vi "dvp Vi Get Frame.vi"(6 "timeout":u32, 7 "piHeight":i32, 9 "piWidth":i32, 10 "pbits":u32(ring) items=["BITS_8", "BITS_10", "BITS_12", "BITS_14", "BITS_16"], 11 "handle":u32) -> (1 "piWidth out":i32, 2 "pbits out":u32(ring) items=["BITS_8", "BITS_10", "BITS_12", "BITS_14", "BITS_16"], 3 "function return":string, 5 "piHeight out":i32)   [LabVIEW 2018, in "LabViewDVPCamera.lvlib"]
doc: "LabviewDvp2Api char* dvpViGetFrame(\n dvpHandle handle,\n dvpBits *pbits,\n dvpInt32 *piWidth,\n dvpInt32 *piHeight,\n dvpUint32 timeout);"
uses:
  LabViewDVPCamera.lvlib
  LabViewDVPCamera/LabViewDVPCamera.dll
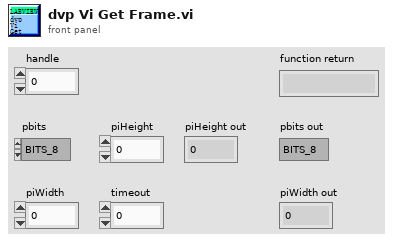
[diagram p1: front panel]
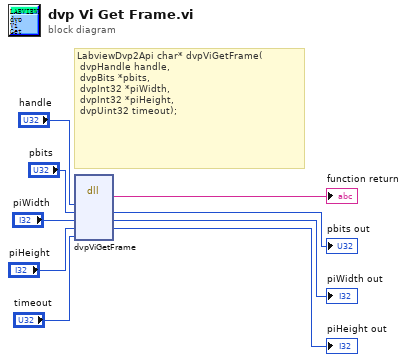
[diagram p0: block diagram]
diagram:
  # "LabviewDvp2Api char* dvpViGetFrame(\n\tdvpHandle handle,\n\tdvpBits *pbits,\n\tdvpInt32 *piWidth,\n\tdvpInt32 *piHeight,\n\tdvpUint32 timeout);"
  n1 = dll-call lib="C:/Program Files (x86)/DVP2 Labview cn 64/Sample/LabViewDVPCamera/LabViewDVPCamera.*" fn="dvpViGetFrame"("handle"="handle", "pbits"="pbits", "piWidth"="piWidth", "piHeight"="piHeight", "timeout"="timeout") -> (→"function return":string, "pbits"=→"pbits out":u32, "piWidth"=→"piWidth out":i32, "piHeight"=→"piHeight out":i32)  [unwired: 5 in, 2 out]
